vi "SeCrTS-DD Queue Data log module.vi"(8 "error in":errorcluster) -> (0 "error out":errorcluster)   [LabVIEW 2022 SP3]
uses:
  Control/SeCrTS-Datalog enumDD.ctl
  e6382295-4c4d-49e8-89a6-fbaf064f03f5.vi
  Globals/SeCrTS-DD globals.vi
panel:
  out "Datalog path":path
  out "x":u32
  out "x-y":dbl
  out "Restart":bool
  out "Log health":bool
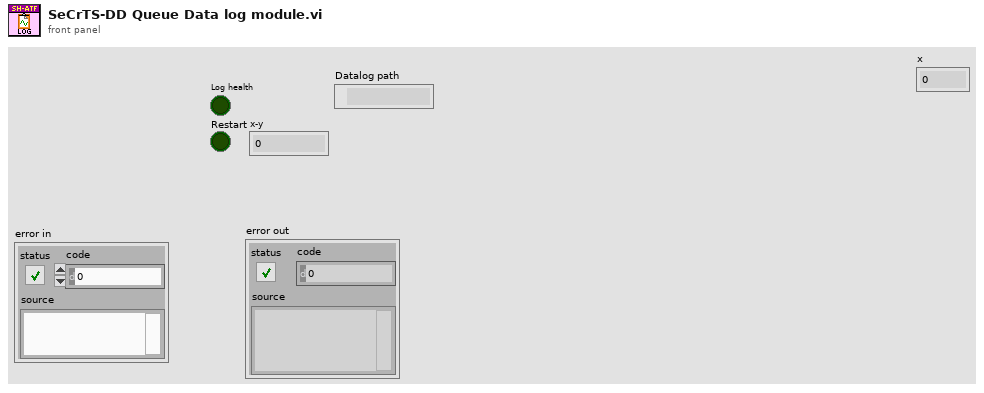
[diagram p1: front panel]
types:
  T1 = cluster{"Log In Progress?":bool, "Log Start Time":timestamp, "Analog Queues":refnum<queue>[], "Digital Queues":refnum<queue>[], "tdms file ref":refnum<k34>}
  T2 = typedef "SeCrTS-Datalog enumDD.ctl" = enum16{"Initialize", "Poll", "Create file", "log Analog", "log Digital", "Flush Queues", "Close file", "Error", "Exit"}
  T3 = enum16{"open", "open or create", "create or replace", "create", "open (read-only)"}
  T4 = cluster{"Datalog path":path, "Configuration path":path, "Signal list path":path, "Sub vi's":path, "Authentication":path}
  T5 = cluster{"Channel names":cluster{"AI_C_Data P":string[], "AI_V_Data P":string[], "AO_Data P":string[], "DO_Data P":string[], "ACC_Data P":string[], "TC Data P":string[], "Drive_A_C":string[], "Drive_A_D":string[], "AI_C_Data S":string[], "DO_Data S":string[]}, "DI Names":cluster{"Di P":string[], "Di S":string[]}}
  T6 = cluster{"AI_C_Data P":string[], "AI_V_Data P":string[], "AO_Data P":string[], "DO_Data P":string[], "ACC_Data P":string[], "TC Data P":string[], "Drive_A_C":string[], "Drive_A_D":string[], "AI_C_Data S":string[], "DO_Data S":string[]}
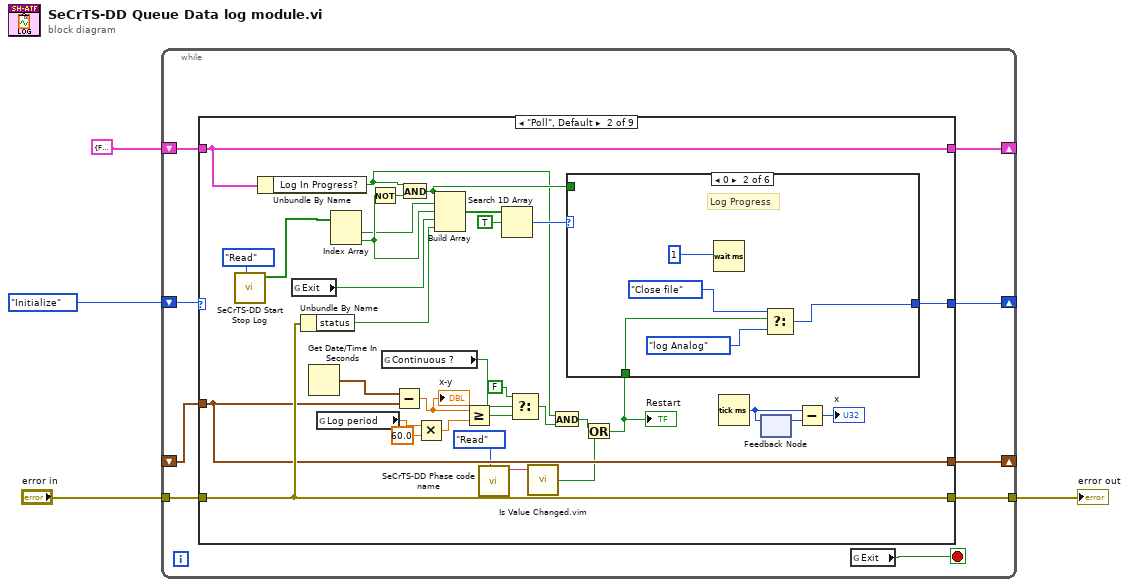
[diagram p0: block diagram]
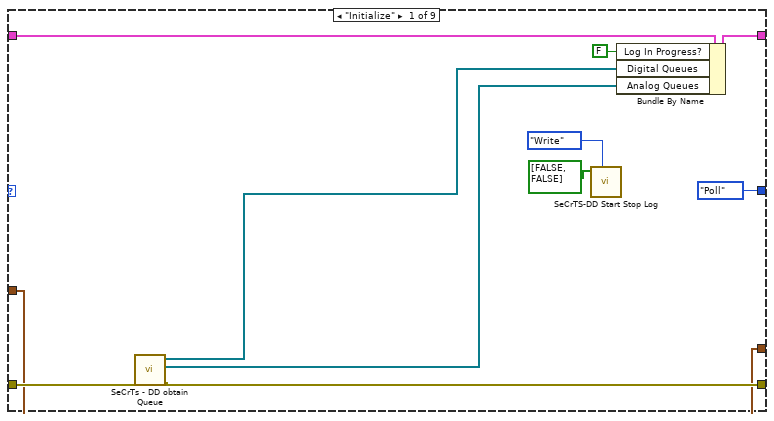
[diagram p2: hidden frame]
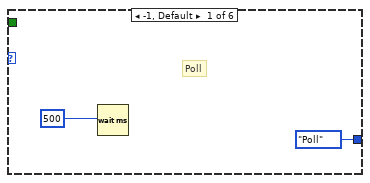
[diagram p3: hidden frame]
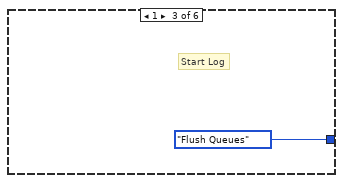
[diagram p4: hidden frame]
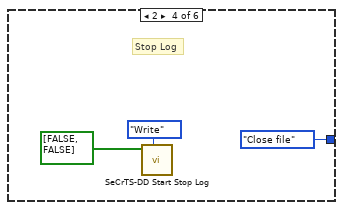
[diagram p5: hidden frame]
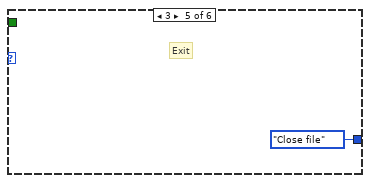
[diagram p6: hidden frame]
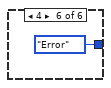
[diagram p7: hidden frame]
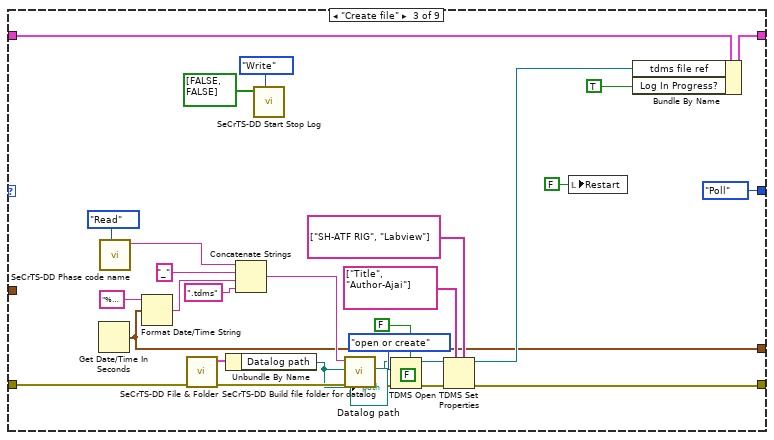
[diagram p8: hidden frame]
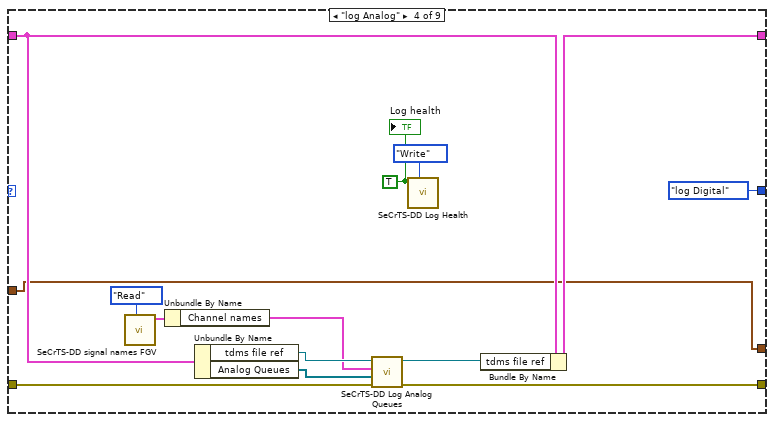
[diagram p9: hidden frame]
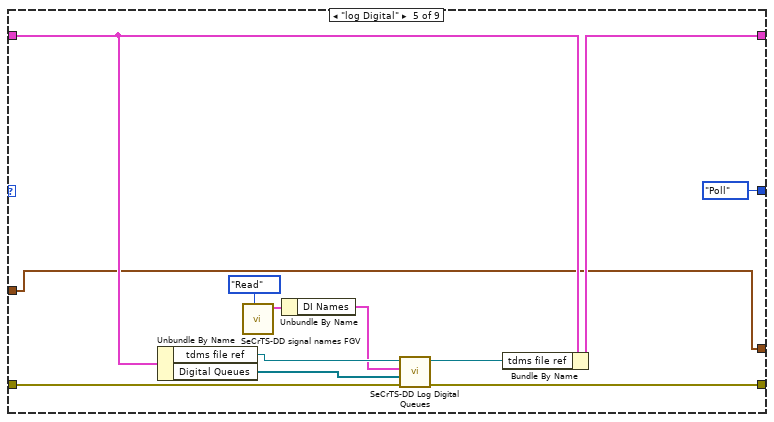
[diagram p10: hidden frame]
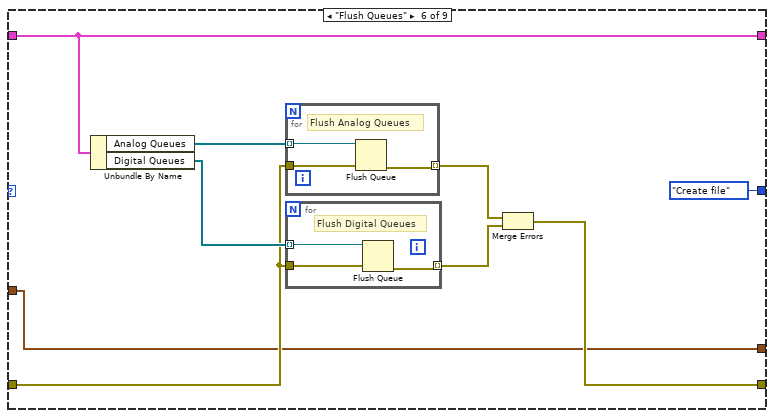
[diagram p11: hidden frame]
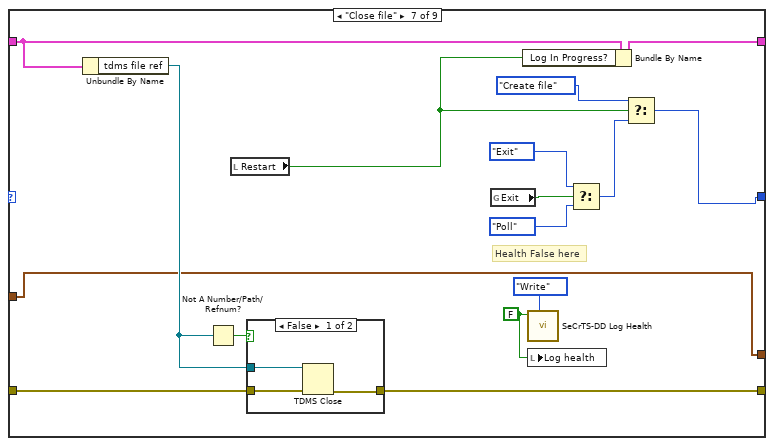
[diagram p12: hidden frame]
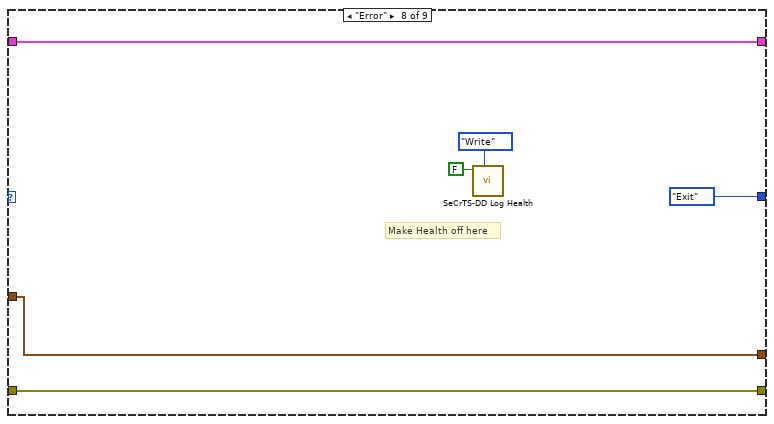
[diagram p14: hidden frame]
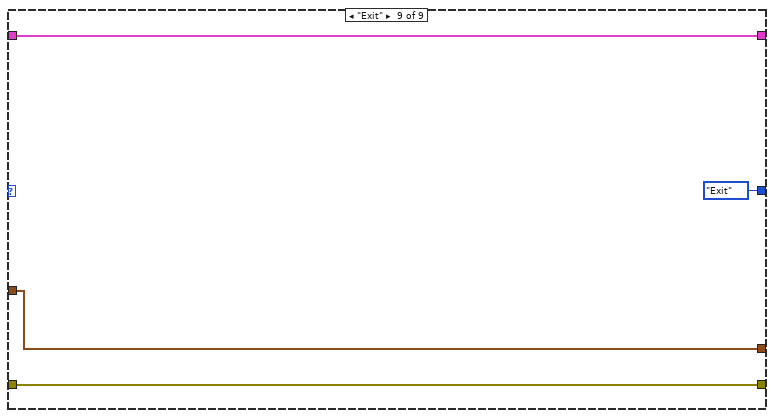
[diagram p15: hidden frame]
diagram:
  n1 = while {
    shift-right: [w8] -> _
    shift-left: SeCrTS-Datalog_enumDD."Initialize" -> [w13]
    shift-right: [w10] -> _
    shift-left: T1 {"Log In Progress?"=FALSE, "Log Start Time"=timestamp(0 s since 1904-01-01), "Analog Queues"=[], "Digital Queues"=[], "tdms file ref"=refnum} -> [w11]
    shift-right: [w5] -> _
    shift-left: _ -> [w6]
    tunnel: "error in" -> [w12]
    tunnel: [w9] -> w1
    stop <- w7 stop-if-true
    n2 = case shown="\"Poll\", Default" w13 {
      tunnel: w12 -> [w23 w51 w94 w110 w124 w130 w152 w164 w169]
      tunnel: w11 -> [w24 w57 w83 w112 w122 w133 w153 w166 w170]
      tunnel: [w22 w57 w82 w107 w119 w133 w154 w166 w170] -> w10
      tunnel: [w18 w51 w79 w109 w123 w127 w151 w164 w169] -> w9
      tunnel: [SeCrTS-Datalog_enumDD."Poll" w52 SeCrTS-Datalog_enumDD."Poll" SeCrTS-Datalog_enumDD."log Digital" SeCrTS-Datalog_enumDD."Poll" SeCrTS-Datalog_enumDD."Create file" w141 SeCrTS-Datalog_enumDD."Exit" SeCrTS-Datalog_enumDD."Exit"] -> w8
      tunnel: w6 -> [w16 w42 _ w100 w114 w126 w145 w161 w167]
      tunnel: [w16 w42 w73 w100 w114 w126 w145 w161 w167] -> w5
      frame "Initialize" {
        n3 = call "SeCrTs - DD obtain Queue.vi"("error in"=w23) -> ("error out"=w18:errorcluster, "AI_V_Data P\nAI_C_Data P\nAO_Data P\nDO_Data P\nACC_Data P\nTC Data P\nDrive_A_C \nDrive_A_D\nAI_C_Data S\nDO_Data S\nAI_V_Rms_P"=w19:refnum<queue>[], "DI P\nDI S"=w20:refnum<queue>[])  [unwired: 8 in]
        n4 = call "SeCrTS-DD Start Stop Log.vi"("Enum"=enum16{"Read", "Write"}."Write", "Start Stop log"=bool[] [FALSE, FALSE]) -> ()  [unwired: 8 in, 2 out]
        n5 = Bundle By Name(cluster=w24, "Log In Progress?"=FALSE, "Digital Queues"=w20, "Analog Queues"=w19) -> (w22:T1)
      }
      frame "Poll", Default {
        n6 = call "SeCrTS-DD Start Stop Log.vi"("Enum"=enum16{"Read", "Write"}."Read") -> ("Start Stop log R"=w38:bool[])  [unwired: 9 in, 1 out]
        n7 = Unbundle By Name(w57) -> ("Log In Progress?"=w33:bool)
        n8 = global read "SeCrTS-DD globals.vi" "Exit"() -> (w47:bool)
        n9 = Unbundle By Name(w51) -> ("status"=w56:bool)
        n10 = Get Date/Time In Seconds() -> (seconds since 1Jan1904=w43:timestamp)
        n11 = global read "SeCrTS-DD globals.vi" "Log period"() -> (w32:dbl)
        n12 = Index Array(array=w38) -> (element #1=w48:bool, element #2=w49:bool)  [unwired: 2 in]
        n13 = Not(x=w49) -> (.not. x?=w50:bool)
        n14 = global read "SeCrTS-DD globals.vi" "Continuous ?"() -> (w37:bool)
        n15 = Subtract(x=w43, y=w42) -> (x-y=w44:dbl)
        "x-y" <- w44
        n16 = And(x=w33, y=w50) -> (x .and. y?=w45:bool)
        n17 = Multiply(x=w32, y=60.0) -> (x*y=w30:dbl)
        n18 = Build Array(w45, w48, w49, w47, w56) -> (w55:bool[])
        n19 = Greater Or Equal?(x=w44, y=w30) -> (x >= y?=w36:bool)
        n20 = call "SeCrTS-DD Phase code name.vi"("Enum"=enum16{"Read", "Write"}."Read") -> ("Phase codeR"=w26:string)  [unwired: 9 in, 1 out]
        n21 = Search 1D Array(1D array=w55, element=TRUE) -> (index of element=w53:i32)  [unwired: 1 in]
        n22 = Select(t=FALSE, s=w37, f=w36) -> (s? t:f=w34:bool)
        n23 = call "Is Value Changed.vim"("value"=w26) -> ("changed or first call?"=w25:bool)
        n24 = And(x=w33, y=w34) -> (x .and. y?=w28:bool)
        n25 = Or(x=w28, y=w25) -> (x .or. y?=w29:bool)
        "Restart" <- w29
        n26 = case shown="0" w53 {
          tunnel: [SeCrTS-Datalog_enumDD."Poll" w61 SeCrTS-Datalog_enumDD."Flush Queues" SeCrTS-Datalog_enumDD."Close file" SeCrTS-Datalog_enumDD."Close file" SeCrTS-Datalog_enumDD."Error"] -> w52
          tunnel: w45 -> [_ _ _ _ _ _]
          tunnel: w29 -> [_ w64 _ _ _ _]
          frame -1, Default {
            # "Poll"
            n27 = Wait (ms)(milliseconds to wait=u32 500 ("millisecond timer value")) -> ()  [unwired: 1 out]
          }
          frame 0 {
            # "Log Progress"
            n28 = Wait (ms)(milliseconds to wait=u32 1 ("millisecond timer value")) -> ()  [unwired: 1 out]
            n29 = Select(t=SeCrTS-Datalog_enumDD."Close file", s=w64, f=SeCrTS-Datalog_enumDD."log Analog") -> (s? t:f=w61:T2)
          }
          frame 1 {
            # "Start Log"
          }
          frame 2 {
            # "Stop Log"
            n30 = call "SeCrTS-DD Start Stop Log.vi"("Enum"=enum16{"Read", "Write"}."Write", "Start Stop log"=bool[] [FALSE, FALSE]) -> ()  [unwired: 8 in, 2 out]
          }
          frame 3 {
            # "Exit"
          }
          frame 4 {
          }
        }
        n31 = Tick Count (ms)() -> (millisecond timer value=w40:u32)
        n32 = feedback #1() -> (w41:u32)  [unwired: 1 in]
        n33 = feedback-in #1(w40) -> ()
        n34 = Subtract(x=w40, y=w41) -> (x-y=→"x":u32)
      }
      frame "Create file" {
        (unwired) FALSE ("disable buffering? (T)")
        n35 = Get Date/Time In Seconds() -> (seconds since 1Jan1904=w73:timestamp)
        n36 = call "SeCrTS-DD Phase code name.vi"("Enum"=enum16{"Read", "Write"}."Read") -> ("Phase codeR"=w74:string)  [unwired: 9 in, 1 out]
        n37 = Format Date/Time String(time format string (%c)="%Y_%b_%d_%Hh_%Mm_%Ssec", seconds (now)=w73) -> (date/time string=w99:string)  [unwired: 1 in]
        n38 = call "SeCrTS-DD File & Folder.vi"("error in (no error)"=w94) -> ("error out"=w93:errorcluster, "File Output"=w92:T4)  [unwired: 9 in]
        n39 = Unbundle By Name(w92) -> ("Datalog path"=w91:path)
        "Datalog path" <- w91
        n40 = Concatenate Strings(w74, "_" ("string"), w99, ".tdms" ("string")) -> (w95:string)
        n41 = call "SeCrTS-DD Start Stop Log.vi"("Enum"=enum16{"Read", "Write"}."Write", "Start Stop log"=bool[] [FALSE, FALSE]) -> ()  [unwired: 8 in, 2 out]
        n42 = call "SeCrTS-DD Build file folder for datalog.vi"("error in (no error)"=w93, "Base Path"=w91, "File Name"=w95) -> ("error out"=w85:errorcluster, "Result File path"=w84:path)  [unwired: 6 in, 1 out]
        n43 = TDMS Open(5:FALSE ("create index file? (T)"), 8:w85, 10:T3."open or create" ("operation (0:open)"), 11:w84) -> (0:w89:errorcluster, 3:w88:refnum<k34>)  [unwired: 3 in]
        n44 = TDMS Set Properties(5:string[] ["SH-ATF RIG", "Labview"] ("property names"), 7:string[] ["Title", "Author-Ajai"] ("property names"), 8:w89, 11:w88) -> (0:w79:errorcluster, 3:w81:refnum<k34>)  [unwired: 4 out]
        n45 = local write "Restart"(FALSE ("Restart")) -> ()
        n46 = Bundle By Name(cluster=w83, "tdms file ref"=w81, "Log In Progress?"=TRUE) -> (w82:T1)
      }
      frame "log Analog" {
        w104 = TRUE ("Log health")
        n47 = call "SeCrTS-DD signal names FGV.vi"("Enum"=enum16{"Read", "Write"}."Read") -> ("Signal names"=w102:T5)  [unwired: 9 in, 1 out]
        n48 = Unbundle By Name(w102) -> ("Channel names"=w101:T6)
        n49 = Unbundle By Name(w112) -> ("tdms file ref"=w108:refnum<k34>, "Analog Queues"=w111:refnum<queue>[])
        n50 = call "SeCrTS-DD Log Analog Queues.vi"("error in"=w110, "AI_V_Data P\nAI_C_Data P\nAO_Data P\nDO_Data P\nACC_Data P\nTC Data P\nDrive_A_C \nDrive_A_D\nAI_C_Data S\nDO_Data S\nAI_V_Rms_P"=w111, "Channel names"=w101, "tdms file in"=w108) -> ("error out"=w109:errorcluster, "tdms ref out"=w106:refnum<k34>)  [unwired: 6 in]
        n51 = call "SeCrTS-DD Log Health.vi"("Enum"=enum16{"Read", "Write"}."Write", "Log health"=w104) -> ()  [unwired: 8 in, 2 out]
        n52 = Bundle By Name(cluster=w112, "tdms file ref"=w106) -> (w107:T1)
        "Log health" <- w104
      }
      frame "log Digital" {
        n53 = Unbundle By Name(w122) -> ("tdms file ref"=w121:refnum<k34>, "Digital Queues"=w120:refnum<queue>[])
        n54 = call "SeCrTS-DD signal names FGV.vi"("Enum"=enum16{"Read", "Write"}."Read") -> ("Signal names"=w116:T5)  [unwired: 9 in, 1 out]
        n55 = Unbundle By Name(w116) -> ("DI Names"=w115:cluster{"Di P":string[], "Di S":string[]})
        n56 = call "SeCrTS-DD Log Digital Queues.vi"("error in"=w124, "DI_queue"=w120, "DI Names 2"=w115, "tdms file in"=w121) -> ("error out"=w123:errorcluster, "tdms file out"=w118:refnum<k34>)  [unwired: 6 in]
        n57 = Bundle By Name(cluster=w122, "tdms file ref"=w118) -> (w119:T1)
      }
      frame "Flush Queues" {
        n58 = Unbundle By Name(w133) -> ("Analog Queues"=w132:refnum<queue>[], "Digital Queues"=w131:refnum<queue>[])
        n59 = for {
          tunnel: w132 -> [w140] mode=indexing
          tunnel: w130 -> [w139]
          tunnel: [w138] -> w129 mode=indexing
          # "Flush Analog Queues"
          n60 = Flush Queue(queue=w140, error in (no error)=w139) -> (error out=w138:errorcluster)  [unwired: 2 out]
        }
        n61 = for {
          tunnel: w131 -> [w137] mode=indexing
          tunnel: w130 -> [w136]
          tunnel: [w135] -> w128 mode=indexing
          # "Flush Digital Queues"
          n62 = Flush Queue(queue=w137, error in (no error)=w136) -> (error out=w135:errorcluster)  [unwired: 2 out]
        }
        n63 = Merge Errors(w129, w128) -> (w127:errorcluster)
      }
      frame "Close file" {
        w146 = FALSE ("Log health")
        # "Health False here"
        n64 = Unbundle By Name(w153) -> ("tdms file ref"=w149:refnum<k34>)
        n65 = Not A Number/Path/Refnum?(number/path/refnum=w149) -> (NaN/Path/Refnum?=w150:bool)
        n66 = local read "Restart"() -> (w144:bool)
        n67 = case shown="False" w150 {
          tunnel: w152 -> [w159 w160]
          tunnel: [w158 w160] -> w151
          tunnel: w149 -> [w157 _]
          frame False {
            n68 = TDMS Close(8:w159, 11:w157) -> (0:w158:errorcluster)  [unwired: 1 out]
          }
          frame True {
          }
        }
        n69 = global read "SeCrTS-DD globals.vi" "Exit"() -> (w147:bool)
        n70 = Bundle By Name(cluster=w153, "Log In Progress?"=w144) -> (w154:T1)
        n71 = call "SeCrTS-DD Log Health.vi"("Enum"=enum16{"Read", "Write"}."Write", "Log health"=w146) -> ()  [unwired: 8 in, 2 out]
        n72 = local write "Log health"(w146) -> ()
        n73 = Select(t=SeCrTS-Datalog_enumDD."Exit", s=w147, f=SeCrTS-Datalog_enumDD."Poll") -> (s? t:f=w142:T2)
        n74 = Select(t=SeCrTS-Datalog_enumDD."Create file", s=w144, f=w142) -> (s? t:f=w141:T2)
      }
      frame "Error" {
        # "Make Health off here"
        n75 = call "SeCrTS-DD Log Health.vi"("Enum"=enum16{"Read", "Write"}."Write", "Log health"=FALSE) -> ()  [unwired: 8 in, 2 out]
      }
      frame "Exit" {
      }
    }
    n76 = global read "SeCrTS-DD globals.vi" "Exit"() -> (w7:bool)
  }
  "error out" <- w1
